vi "Document.vi"   [LabVIEW 2018, in "Scripts.lvlib"]
uses:
  Scripts.lvlib
  <vilib>/Field R&D Services/Labricator/Toolkit/Labricator.lvlib
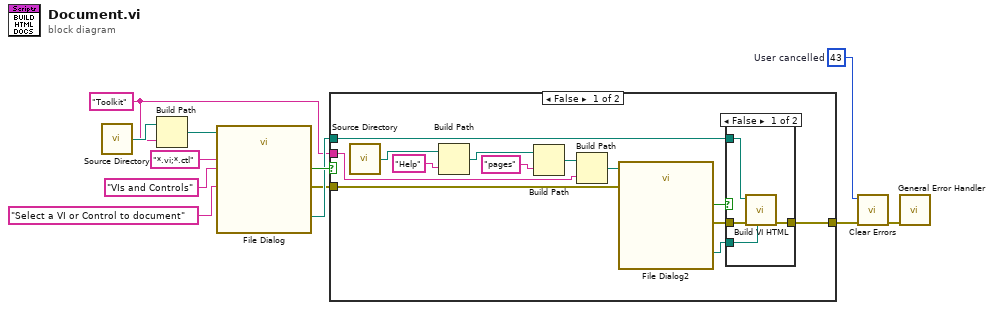
[diagram p0: block diagram]
diagram:
  w4 = 43  # User cancelled
  w1 = "Toolkit" ("name or relative path")
  n1 = call <vilib>:"Source Directory.vi"() -> ("Source Directory"=w6:path)
  n2 = Build Path(base path=w6, name or relative path=w1) -> (appended path=w10:path)
  n3 = call "File Dialog"("start path"=w10, "prompt"="Select a VI or Control to document", "pattern (all files)"="*.vi;*.ctl", "pattern label"="VIs and Controls") -> ("selected path"=w11:path, "cancelled"=w12:bool, "error out"=w3:errorcluster)  [unwired: 8 in, 1 out]
  n4 = case shown="False" w12 {
    tunnel: w3 -> [w24 w31]
    tunnel: w11 -> [w25 _]
    tunnel: [w20 w31] -> w2
    tunnel: w1 -> [w14 _]
    frame False {
      n5 = call <vilib>:"Source Directory.vi"() -> ("Source Directory"=w19:path)
      n6 = Build Path(base path=w19, name or relative path="Help") -> (appended path=w17:path)
      n7 = Build Path(base path=w17, name or relative path="pages") -> (appended path=w15:path)
      n8 = Build Path(base path=w15, name or relative path=w14) -> (appended path=w13:path)
      n9 = call "File Dialog2"("start path"=w13, "error in"=w24) -> ("selected path"=w22:path, "cancelled"=w21:bool, "error out"=w23:errorcluster)  [unwired: 10 in, 1 out]
      n10 = case shown="False" w21 {
        tunnel: [w29 w30] -> w20
        tunnel: w25 -> [w28 _]
        tunnel: w23 -> [w27 w30]
        tunnel: w22 -> [w26 _]
        frame False {
          n11 = call "Build VI HTML.vi"("Destination"=w26, "Error In"=w27, "VI"=w28) -> ("Error Out"=w29:errorcluster)  [unwired: 8 in]
        }
        frame True {
        }
      }
    }
    frame True {
    }
  }
  n12 = call <vilib>:"Clear Errors.vi"("error in (no error)"=w2, "specific error code to clear (0: all)"=w4) -> ("error out"=w5:errorcluster)  [unwired: 4 in, 1 out]
  n13 = call <vilib>:"General Error Handler.vi"("error in (no error)"=w5) -> ()  [unwired: 10 in, 5 out]
